vi "Run Optimiser.vi"(7 "Analysis Framework":refnum<class "Analysis Framework.lvclass">, 8 "error in (no error)":errorcluster, 11 "Optimiser Cell in":refnum<class "Optimiser Cell.lvclass">) -> (0 "error out":errorcluster, 3 "Optimiser Cell out":refnum<class "Optimiser Cell.lvclass">, 4 "Optimiser Finished":bool)   [LabVIEW 2020, in "CIRCUS_uServices.lvlib" / "Run Utilities.lvlib" / "Optimiser Cell.lvclass"]
doc: "This VI calls the optimiser (from the Analysis Framework) and updates the parameters of the Run Instance based on the suggestion from the optimiser."
uses:
  Optimiser Cell.lvclass
  Optimiser Cell.lvclass/Optimiser Cell.ctl
  C:/Users/marco/Documents/GitHub_Lab/CIRCUS/CIRCUS uServices et al/Run Utilities/Cell/Schedule Cell.lvclass
  C:/Users/marco/Documents/GitHub_Lab/CIRCUS/CIRCUS uServices et al/Run Utilities/Optimiser Cell/Optimiser Cell.lvclass
  Analysis Framework/Analysis Framework.lvclass
  TALOS/TALOS_PPL.lvlibp
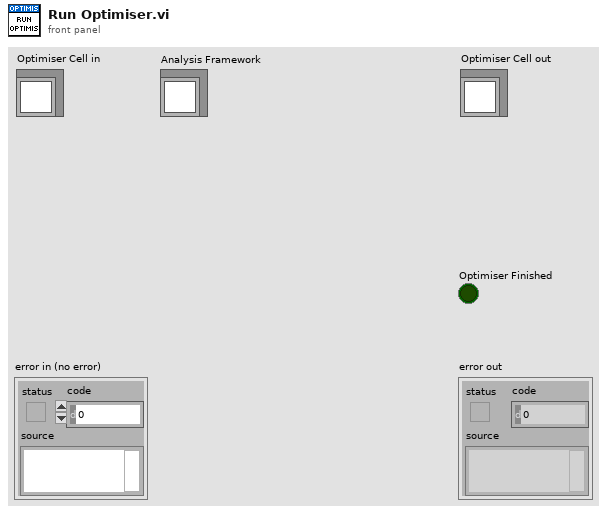
[diagram p1: front panel]
types:
  T1 = typedef "Run Utilities.lvlib/Optimiser Cell.lvclass/Optimise parameter - numeric.ctl" = cluster{"Name":string, "Start value":dbl, "From":dbl, "To":dbl, "dtype":enum16{"INT", "DBL"}}
  T2 = typedef "Run Utilities.lvlib/Optimiser Cell.lvclass/Optimise parameter - string.ctl" = cluster{"Name":string, "Start value":string, "Options":string[]}
  T3 = typedef "Run Utilities.lvlib/Optimiser Cell.lvclass/Optimiser Results.ctl" = cluster{"Array of Parameters":T4[], "Target":string}
  T4 = typedef "Analysis Framework.lvclass/Name with value pair.ctl" = cluster{"Name":string, "Value":string}
  T5 = typedef "Run Utilities.lvlib/Optimiser Cell.lvclass/Optimisation Strategy.ctl" = enum16{"Maximize", "Minimize", "Value"}
  T6 = cluster{"Number of Exploration Runs":i32, "Parameters - numeric":T1[], "Parameters - string":T2[], "History":T3[], "Optimisation Strategy":T5, "Value":dbl}
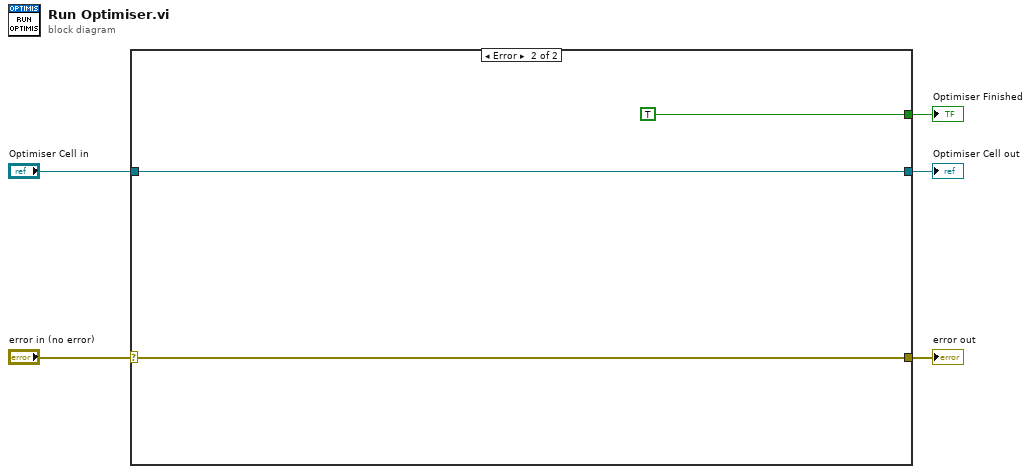
[diagram p0: block diagram]
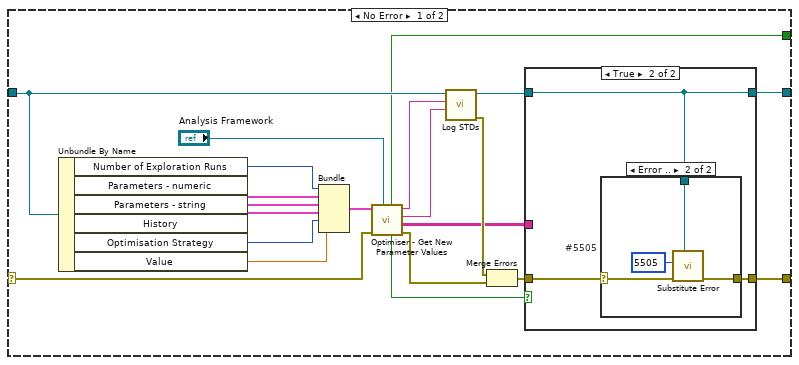
[diagram p2: hidden frame]
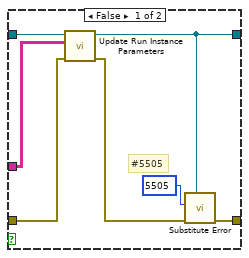
[diagram p3: hidden frame]
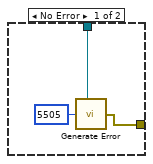
[diagram p4: hidden frame]
diagram:
  n1 = case shown="Error" "error in (no error)" {
    selector: "error in (no error)" -> [w12 w46]
    tunnel: [w25 w46] -> w4
    tunnel: [w26 w45] -> w1
    tunnel: "Optimiser Cell in" -> [w22 w45]
    tunnel: [w9 TRUE ("Optimise Finished")] -> w2
    frame No Error {
      n2 = Unbundle By Name(w22) -> ("Number of Exploration Runs"=w19:i32, "Parameters - numeric"=w15:T1[], "Parameters - string"=w14:T2[], "History"=w18:T3[], "Optimisation Strategy"=w17:T5, "Value"=w16:dbl)
      n3 = Bundle("Number of Exploration Runs"=w19, "Parameters - numeric"=w15, "Parameters - string"=w14, "History"=w18, "Optimisation Strategy"=w17, "Value"=w16) -> (w13:T6)  [unwired: 1 in]
      n4 = call-dynamic "Optimiser - Get New Parameter Values.vi"("Analysis Framework in"="Analysis Framework", "error in (no error)"=w12, "optimisation cluster"=w13) -> ("error out"=w11:errorcluster, "Parameters"=w6:string[][], "standard error"=w7:string, "standard output"=w8:string, "Error"=w10:bool, "Optimise Finished"=w9:bool)  [unwired: 3 in]
      n5 = call-dynamic "Log STDs.vi"("StdErr"=w7, "StdOut"=w8, "Run Optimiser in"=w22) -> ("error out"=w21:errorcluster, "Run Optimiser out"=w23:refnum<class "Optimiser Cell.lvclass">)  [unwired: 7 in]
      n6 = Merge Errors(w21, w11) -> (w24:errorcluster)
      n7 = case shown="True" w10 {
        tunnel: w23 -> [w30 w35]
        tunnel: [w31 w35] -> w26
        tunnel: [w32 w34] -> w25
        tunnel: w24 -> [w28 w36]
        tunnel: w6 -> [w29 _]
        frame False {
          # "#5505"
          n8 = call-dynamic "Update Run Instance Parameters.vi"("error in (no error)"=w28, "Parameters"=w29, "Optimiser Cell in"=w30) -> ("error out"=w27:errorcluster, "Optimiser Cell out"=w31:refnum<class "Optimiser Cell.lvclass">)  [unwired: 7 in]
          n9 = call "Substitute Error.vi"("LabVIEW Object"=w31, "error in (no error)"=w27, "Error Code"=5505) -> ("error out"=w32:errorcluster)  [unwired: 8 in]
        }
        frame True {
          n10 = case "#5505" shown="Error .." w36 {
            selector: w36 -> [_ w41]
            tunnel: w35 -> [w39 w43]
            tunnel: [w37 w42] -> w34
            frame No Error {
              n11 = call "Generate Error.vi"("Class"=w39, "Error Code"=5505) -> ("error out"=w37:errorcluster)  [unwired: 5 in]
            }
            frame Error {
              n12 = call "Substitute Error.vi"("LabVIEW Object"=w43, "error in (no error)"=w41, "Error Code"=5505) -> ("error out"=w42:errorcluster)  [unwired: 8 in]
            }
          }
        }
      }
    }
    frame Error {
    }
  }
  "error out" <- w4
  "Optimiser Cell out" <- w1
  "Optimiser Finished" <- w2
